vi "Voltage.vi"() -> ()   [LabVIEW 2013]
panel:
  out "Voltage":dbl
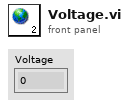
[diagram p1: front panel]
diagram:
